vi "_UpdateCalMethod.vi"(4 "Model Name":T1=enum."IONICS 3Q 210", 5 "UsingESI1":bool=TRUE, 6 "error in (no error)":errorcluster, 7 "Q1/Q2":string="Q1", 8 "CalOption":enum32{"Positive", "Negative"}(radio), 9 "Method":T2={"Lenses"=[{"Scan Type"=0, "Scans"=1000, "Time 1"=0.0, "Time 2"=5.0, "Value 1"=400.0, "Value 2"=400.0, "Step Size"=1.0}, {"Scan Type"=0, "Scans"=1, "Time 1"=1.0, "Time 2"=1.0, "Value 1"=600.0, "Value 2"=600.0, "Step Size"=1.0}, {"Scan Type"=0, "Scans"=1, "Time 1"=1.0, "Time 2"=1.0, "Value 1"=32000.0, "Value 2"=32000.0, "Step Size"=1.0}, {"Scan Type"=0, "Scans"=1, "Time 1"=1.0, "Time 2"=1.0, "Value 1"=400.0, "Value 2"=400.0, "Step Size"=1.0}, {"Scan Type"=0, "Scans"=1, "Time 1"=1.0, "Time 2"=1.0, "Value 1"=600.0, "Value 2"=600.0, "Step Size"=1.0}, {"Scan Type"=0, "Scans"=1, "Time 1"=1.0, "Time 2"=1.0, "Value 1"=32000.0, "Value 2"=32000.0, "Step Size"=1.0}, {"Scan Type"=0, "Scans"=1, "Time 1"=1.0, "Time 2"=1.0, "Value 1"=500.0, "Value 2"=400.0, "Step Size"=1.0}, {"Scan Type"=0, "Scans"=1, "Time 1"=1.0, "Time 2"=1.0, "Value 1"=70.0, "Value 2"=80.0, "Step Size"=1.0}, {"Scan Type"=0, "Scans"=1, "Time 1"=1.0, "Time 2"=1.0, "Value 1"=80.0, "Value 2"=80.0, "Step Size"=1.0}, {"Scan Type"=0, "Scans"=1, "Time 1"=1.0, "Time 2"=1.0, "Value 1"=-1.0, "Value 2"=100.0, "Step Size"=1.0}, {"Scan Type"=0, "Scans"=1, "Time 1"=1.0, "Time 2"=1.0, "Value 1"=-2.0, "Value 2"=100.0, "Step Size"=1.0}, {"Scan Type"=0, "Scans"=1, "Time 1"=1.0, "Time 2"=1.0, "Value 1"=-3.0, "Value 2"=100.0, "Step Size"=1.0}, {"Scan Type"=0, "Scans"=1, "Time 1"=1.0, "Time 2"=1.0, "Value 1"=-4.0, "Value 2"=100.0, "Step Size"=1.0}, {"Scan Type"=0, "Scans"=1, "Time 1"=1.0, "Time 2"=1.0, "Value 1"=-15.0, "Value 2"=100.0, "Step Size"=1.0}, {"Scan Type"=0, "Scans"=1, "Time 1"=1.0, "Time 2"=1.0, "Value 1"=-4.5, "Value 2"=-9.0, "Step Size"=1.0}, {"Scan Type"=0, "Scans"=1, "Time 1"=1.0, "Time 2"=1.0, "Value 1"=0.0, "Value 2"=100.0, "Step Size"=1.0}, {"Scan Type"=0, "Scans"=1, "Time 1"=1.0, "Time 2"=1.0, "Value 1"=-100.0, "Value 2"=100.0, "Step Size"=1.0}, {"Scan Type"=0, "Scans"=1, "Time 1"=1.0, "Time 2"=1.0, "Value 1"=-50.0, "Value 2"=100.0, "Step Size"=1.0}, {"Scan Type"=0, "Scans"=1, "Time 1"=1.0, "Time 2"=1.0, "Value 1"=100.0, "Value 2"=100.0, "Step Size"=1.0}, {"Scan Type"=0, "Scans"=1, "Time 1"=1.0, "Time 2"=1.0, "Value 1"=-51.0, "Value 2"=100.0, "Step Size"=1.0}, {"Scan Type"=0, "Scans"=1, "Time 1"=1.0, "Time 2"=1.0, "Value 1"=-62.0, "Value 2"=100.0, "Step Size"=1.0}, {"Scan Type"=0, "Scans"=1, "Time 1"=1.0, "Time 2"=1.0, "Value 1"=-52.0, "Value 2"=-150.0, "Step Size"=1.0}, {"Scan Type"=0, "Scans"=1, "Time 1"=1.0, "Time 2"=1.0, "Value 1"=-100.0, "Value 2"=-200.0, "Step Size"=1.0}, {"Scan Type"=0, "Scans"=1, "Time 1"=1.0, "Time 2"=1.0, "Value 1"=15.0, "Value 2"=50.0, "Step Size"=1.0}, {"Scan Type"=0, "Scans"=1, "Time 1"=1.0, "Time 2"=1.0, "Value 1"=2000.0, "Value 2"=500.0, "Step Size"=1.0}, {"Scan Type"=0, "Scans"=1, "Time 1"=1.0, "Time 2"=1.0, "Value 1"=5500.0, "Value 2"=1000.0, "Step Size"=1.0}, {"Scan Type"=0, "Scans"=1, "Time 1"=1.0, "Time 2"=1.0, "Value 1"=420.0, "Value 2"=420.0, "Step Size"=1.0}, {"Scan Type"=0, "Scans"=1, "Time 1"=1.0, "Time 2"=1.0, "Value 1"=-420.0, "Value 2"=-420.0, "Step Size"=1.0}, {"Scan Type"=0, "Scans"=1, "Time 1"=1.0, "Time 2"=1.0, "Value 1"=420.0, "Value 2"=420.0, "Step Size"=1.0}, {"Scan Type"=0, "Scans"=1, "Time 1"=1.0, "Time 2"=1.0, "Value 1"=-420.0, "Value 2"=-420.0, "Step Size"=1.0}, {"Scan Type"=0, "Scans"=1, "Time 1"=1.0, "Time 2"=1.0, "Value 1"=600.0, "Value 2"=600.0, "Step Size"=1.0}, {"Scan Type"=0, "Scans"=1, "Time 1"=1.0, "Time 2"=1.0, "Value 1"=-600.0, "Value 2"=600.0, "Step Size"=1.0}, {"Scan Type"=0, "Scans"=1, "Time 1"=1.0, "Time 2"=1.0, "Value 1"=80.0, "Value 2"=0.9, "Step Size"=1.0}, {"Scan Type"=0, "Scans"=1, "Time 1"=1.0, "Time 2"=1.0, "Value 1"=90.0, "Value 2"=0.0, "Step Size"=1.0}, {"Scan Type"=0, "Scans"=1, "Time 1"=1.0, "Time 2"=1.0, "Value 1"=0.0, "Value 2"=0.0, "Step Size"=1.0}, {"Scan Type"=0, "Scans"=1, "Time 1"=1.0, "Time 2"=1.0, "Value 1"=0.0, "Value 2"=0.0, "Step Size"=1.0}, {"Scan Type"=0, "Scans"=1, "Time 1"=1.0, "Time 2"=1.0, "Value 1"=0.0, "Value 2"=0.0, "Step Size"=1.0}, {"Scan Type"=0, "Scans"=1, "Time 1"=1.0, "Time 2"=1.0, "Value 1"=0.0, "Value 2"=0.0, "Step Size"=1.0}, {"Scan Type"=0, "Scans"=1, "Time 1"=1.0, "Time 2"=1.0, "Value 1"=500.0, "Value 2"=0.0, "Step Size"=1.0}, {"Scan Type"=0, "Scans"=1, "Time 1"=1.0, "Time 2"=1.0, "Value 1"=0.0, "Value 2"=0.0, "Step Size"=1.0}, {"Scan Type"=0, "Scans"=1, "Time 1"=1.0, "Time 2"=1.0, "Value 1"=5850.0, "Value 2"=0.0, "Step Size"=1.0}, {"Scan Type"=0, "Scans"=1, "Time 1"=1.0, "Time 2"=1.0, "Value 1"=0.0, "Value 2"=0.0, "Step Size"=1.0}, {"Scan Type"=0, "Scans"=1, "Time 1"=1.0, "Time 2"=1.0, "Value 1"=1000.0, "Value 2"=0.0, "Step Size"=1.0}, {"Scan Type"=0, "Scans"=1, "Time 1"=1.0, "Time 2"=1.0, "Value 1"=320.0, "Value 2"=0.0, "Step Size"=1.0}, {"Scan Type"=0, "Scans"=1, "Time 1"=1.0, "Time 2"=1.0, "Value 1"=0.0, "Value 2"=0.0, "Step Size"=1.0}, {"Scan Type"=0, "Scans"=1, "Time 1"=1.0, "Time 2"=1.0, "Value 1"=0.0, "Value 2"=0.0, "Step Size"=1.0}], "Mass Ranges"=[{"Start"=54.0, "Stop"=64.0, "Step Size"=0.1, "Steps"=101, "Dwell"=10.0, "Parameters"=[], "Res"=1}, {"Start"=170.0, "Stop"=180.0, "Step Size"=0.1, "Steps"=101, "Dwell"=10.0, "Parameters"=[], "Res"=1}, {"Start"=611.0, "Stop"=621.0, "Step Size"=0.1, "Steps"=101, "Dwell"=10.0, "Parameters"=[], "Res"=1}, {"Start"=902.0, "Stop"=912.0, "Step Size"=0.1, "Steps"=101, "Dwell"=10.0, "Parameters"=[], "Res"=1}, {"Start"=1250.0, "Stop"=1260.0, "Step Size"=0.1, "Steps"=101, "Dwell"=10.0, "Parameters"=[], "Res"=1}, {"Start"=1540.0, "Stop"=1550.0, "Step Size"=0.1, "Steps"=101, "Dwell"=10.0, "Parameters"=[], "Res"=1}, {"Start"=1773.0, "Stop"=1783.0, "Step Size"=0.1, "Steps"=101, "Dwell"=10.0, "Parameters"=[], "Res"=1}, {"Start"=2005.0, "Stop"=2015.0, "Step Size"=0.1, "Steps"=101, "Dwell"=10.0, "Parameters"=[], "Res"=1}], "Acquire"=FALSE, "MCA"=FALSE, "Q1DC EN"=FALSE, "Q1 POL"=FALSE, "Q3 POL"=FALSE, "Q1 RF  EN"=TRUE, "Averaging"=FALSE, "Log Scale"=FALSE, "CPS"=TRUE, "Unit"=FALSE, "Data Path"=path "", "Run Mode"=enum."Q1 Scan", "Fixed Mass (amu)"=609.2, "Q3DC EN"=FALSE, "Q3 RF  EN"=TRUE, "Negative"=FALSE} {"Mass Ranges"."Res" items=["High/High", "Medium/Medium", "Low/Low", "High/Medium", "High/Low", "Medium/High", "Medium/Low", "Low/High", "Low/Medium"]}) -> (0 "error out":errorcluster, 3 "MethodOut":T2={"Lenses"=[{"Scan Type"=0, "Scans"=1000, "Time 1"=0.0, "Time 2"=5.0, "Value 1"=400.0, "Value 2"=400.0, "Step Size"=1.0}, {"Scan Type"=0, "Scans"=1, "Time 1"=1.0, "Time 2"=1.0, "Value 1"=600.0, "Value 2"=600.0, "Step Size"=1.0}, {"Scan Type"=0, "Scans"=1, "Time 1"=1.0, "Time 2"=1.0, "Value 1"=32000.0, "Value 2"=32000.0, "Step Size"=1.0}, {"Scan Type"=0, "Scans"=1, "Time 1"=1.0, "Time 2"=1.0, "Value 1"=400.0, "Value 2"=400.0, "Step Size"=1.0}, {"Scan Type"=0, "Scans"=1, "Time 1"=1.0, "Time 2"=1.0, "Value 1"=600.0, "Value 2"=600.0, "Step Size"=1.0}, {"Scan Type"=0, "Scans"=1, "Time 1"=1.0, "Time 2"=1.0, "Value 1"=32000.0, "Value 2"=32000.0, "Step Size"=1.0}, {"Scan Type"=0, "Scans"=1, "Time 1"=1.0, "Time 2"=1.0, "Value 1"=500.0, "Value 2"=400.0, "Step Size"=1.0}, {"Scan Type"=0, "Scans"=1, "Time 1"=1.0, "Time 2"=1.0, "Value 1"=70.0, "Value 2"=80.0, "Step Size"=1.0}, {"Scan Type"=0, "Scans"=1, "Time 1"=1.0, "Time 2"=1.0, "Value 1"=80.0, "Value 2"=80.0, "Step Size"=1.0}, {"Scan Type"=0, "Scans"=1, "Time 1"=1.0, "Time 2"=1.0, "Value 1"=-1.0, "Value 2"=100.0, "Step Size"=1.0}, {"Scan Type"=0, "Scans"=1, "Time 1"=1.0, "Time 2"=1.0, "Value 1"=-2.0, "Value 2"=100.0, "Step Size"=1.0}, {"Scan Type"=0, "Scans"=1, "Time 1"=1.0, "Time 2"=1.0, "Value 1"=-3.0, "Value 2"=100.0, "Step Size"=1.0}, {"Scan Type"=0, "Scans"=1, "Time 1"=1.0, "Time 2"=1.0, "Value 1"=-4.0, "Value 2"=100.0, "Step Size"=1.0}, {"Scan Type"=0, "Scans"=1, "Time 1"=1.0, "Time 2"=1.0, "Value 1"=-15.0, "Value 2"=100.0, "Step Size"=1.0}, {"Scan Type"=0, "Scans"=1, "Time 1"=1.0, "Time 2"=1.0, "Value 1"=-4.5, "Value 2"=-9.0, "Step Size"=1.0}, {"Scan Type"=0, "Scans"=1, "Time 1"=1.0, "Time 2"=1.0, "Value 1"=0.0, "Value 2"=100.0, "Step Size"=1.0}, {"Scan Type"=0, "Scans"=1, "Time 1"=1.0, "Time 2"=1.0, "Value 1"=-100.0, "Value 2"=100.0, "Step Size"=1.0}, {"Scan Type"=0, "Scans"=1, "Time 1"=1.0, "Time 2"=1.0, "Value 1"=-50.0, "Value 2"=100.0, "Step Size"=1.0}, {"Scan Type"=0, "Scans"=1, "Time 1"=1.0, "Time 2"=1.0, "Value 1"=100.0, "Value 2"=100.0, "Step Size"=1.0}, {"Scan Type"=0, "Scans"=1, "Time 1"=1.0, "Time 2"=1.0, "Value 1"=-51.0, "Value 2"=100.0, "Step Size"=1.0}, {"Scan Type"=0, "Scans"=1, "Time 1"=1.0, "Time 2"=1.0, "Value 1"=-62.0, "Value 2"=100.0, "Step Size"=1.0}, {"Scan Type"=0, "Scans"=1, "Time 1"=1.0, "Time 2"=1.0, "Value 1"=-52.0, "Value 2"=-150.0, "Step Size"=1.0}, {"Scan Type"=0, "Scans"=1, "Time 1"=1.0, "Time 2"=1.0, "Value 1"=-100.0, "Value 2"=-200.0, "Step Size"=1.0}, {"Scan Type"=0, "Scans"=1, "Time 1"=1.0, "Time 2"=1.0, "Value 1"=15.0, "Value 2"=50.0, "Step Size"=1.0}, {"Scan Type"=0, "Scans"=1, "Time 1"=1.0, "Time 2"=1.0, "Value 1"=2000.0, "Value 2"=500.0, "Step Size"=1.0}, {"Scan Type"=0, "Scans"=1, "Time 1"=1.0, "Time 2"=1.0, "Value 1"=5500.0, "Value 2"=1000.0, "Step Size"=1.0}, {"Scan Type"=0, "Scans"=1, "Time 1"=1.0, "Time 2"=1.0, "Value 1"=420.0, "Value 2"=420.0, "Step Size"=1.0}, {"Scan Type"=0, "Scans"=1, "Time 1"=1.0, "Time 2"=1.0, "Value 1"=-420.0, "Value 2"=-420.0, "Step Size"=1.0}, {"Scan Type"=0, "Scans"=1, "Time 1"=1.0, "Time 2"=1.0, "Value 1"=420.0, "Value 2"=420.0, "Step Size"=1.0}, {"Scan Type"=0, "Scans"=1, "Time 1"=1.0, "Time 2"=1.0, "Value 1"=-420.0, "Value 2"=-420.0, "Step Size"=1.0}, {"Scan Type"=0, "Scans"=1, "Time 1"=1.0, "Time 2"=1.0, "Value 1"=600.0, "Value 2"=600.0, "Step Size"=1.0}, {"Scan Type"=0, "Scans"=1, "Time 1"=1.0, "Time 2"=1.0, "Value 1"=-600.0, "Value 2"=600.0, "Step Size"=1.0}, {"Scan Type"=0, "Scans"=1, "Time 1"=1.0, "Time 2"=1.0, "Value 1"=80.0, "Value 2"=0.9, "Step Size"=1.0}, {"Scan Type"=0, "Scans"=1, "Time 1"=1.0, "Time 2"=1.0, "Value 1"=90.0, "Value 2"=0.0, "Step Size"=1.0}, {"Scan Type"=0, "Scans"=1, "Time 1"=1.0, "Time 2"=1.0, "Value 1"=0.0, "Value 2"=0.0, "Step Size"=1.0}, {"Scan Type"=0, "Scans"=1, "Time 1"=1.0, "Time 2"=1.0, "Value 1"=0.0, "Value 2"=0.0, "Step Size"=1.0}, {"Scan Type"=0, "Scans"=1, "Time 1"=1.0, "Time 2"=1.0, "Value 1"=0.0, "Value 2"=0.0, "Step Size"=1.0}, {"Scan Type"=0, "Scans"=1, "Time 1"=1.0, "Time 2"=1.0, "Value 1"=0.0, "Value 2"=0.0, "Step Size"=1.0}, {"Scan Type"=0, "Scans"=1, "Time 1"=1.0, "Time 2"=1.0, "Value 1"=500.0, "Value 2"=0.0, "Step Size"=1.0}, {"Scan Type"=0, "Scans"=1, "Time 1"=1.0, "Time 2"=1.0, "Value 1"=0.0, "Value 2"=0.0, "Step Size"=1.0}, {"Scan Type"=0, "Scans"=1, "Time 1"=1.0, "Time 2"=1.0, "Value 1"=5850.0, "Value 2"=0.0, "Step Size"=1.0}, {"Scan Type"=0, "Scans"=1, "Time 1"=1.0, "Time 2"=1.0, "Value 1"=0.0, "Value 2"=0.0, "Step Size"=1.0}, {"Scan Type"=0, "Scans"=1, "Time 1"=1.0, "Time 2"=1.0, "Value 1"=1000.0, "Value 2"=0.0, "Step Size"=1.0}, {"Scan Type"=0, "Scans"=1, "Time 1"=1.0, "Time 2"=1.0, "Value 1"=320.0, "Value 2"=0.0, "Step Size"=1.0}, {"Scan Type"=0, "Scans"=1, "Time 1"=1.0, "Time 2"=1.0, "Value 1"=0.0, "Value 2"=0.0, "Step Size"=1.0}, {"Scan Type"=0, "Scans"=1, "Time 1"=1.0, "Time 2"=1.0, "Value 1"=0.0, "Value 2"=0.0, "Step Size"=1.0}], "Mass Ranges"=[{"Start"=54.0, "Stop"=64.0, "Step Size"=0.1, "Steps"=101, "Dwell"=10.0, "Parameters"=[], "Res"=1}, {"Start"=170.0, "Stop"=180.0, "Step Size"=0.1, "Steps"=101, "Dwell"=10.0, "Parameters"=[], "Res"=1}, {"Start"=611.0, "Stop"=621.0, "Step Size"=0.1, "Steps"=101, "Dwell"=10.0, "Parameters"=[], "Res"=1}, {"Start"=902.0, "Stop"=912.0, "Step Size"=0.1, "Steps"=101, "Dwell"=10.0, "Parameters"=[], "Res"=1}, {"Start"=1250.0, "Stop"=1260.0, "Step Size"=0.1, "Steps"=101, "Dwell"=10.0, "Parameters"=[], "Res"=1}, {"Start"=1540.0, "Stop"=1550.0, "Step Size"=0.1, "Steps"=101, "Dwell"=10.0, "Parameters"=[], "Res"=1}, {"Start"=1773.0, "Stop"=1783.0, "Step Size"=0.1, "Steps"=101, "Dwell"=10.0, "Parameters"=[], "Res"=1}, {"Start"=2005.0, "Stop"=2015.0, "Step Size"=0.1, "Steps"=101, "Dwell"=10.0, "Parameters"=[], "Res"=1}], "Acquire"=FALSE, "MCA"=FALSE, "Q1DC EN"=FALSE, "Q1 POL"=FALSE, "Q3 POL"=FALSE, "Q1 RF  EN"=TRUE, "Averaging"=FALSE, "Log Scale"=FALSE, "CPS"=TRUE, "Unit"=FALSE, "Data Path"=path "", "Run Mode"=enum."Q1 Scan", "Fixed Mass (amu)"=609.2, "Q3DC EN"=FALSE, "Q3 RF  EN"=TRUE, "Negative"=FALSE} {"Mass Ranges"."Res" items=["High/High", "Medium/Medium", "Low/Low", "High/Medium", "High/Low", "Medium/High", "Medium/Low", "Low/High", "Low/Medium"]})   [LabVIEW 2012]
uses:
  Type/_GUI Method.ctl
  Type/_Lens Property.ctl
  Type/_Mass Range Property.ctl
  Type/_Mass Range Parameters.ctl
  Type/_RT Res Type.ctl
  Type/_Run Mode.ctl
  Type/_Instrument Model.ctl
panel:
  in  "CurrentDV":dbl=2000.0
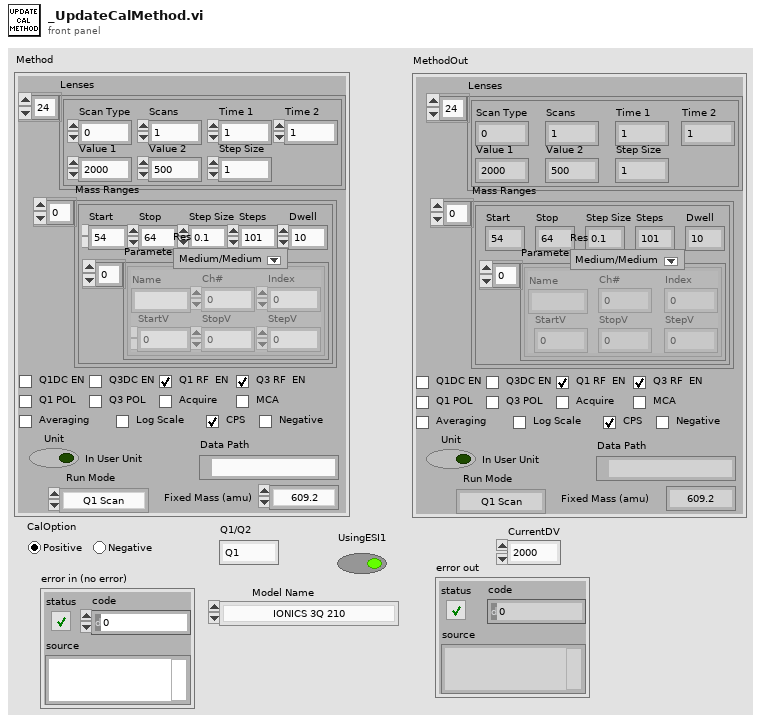
[diagram p1: front panel]
types:
  T1 = typedef "_Instrument Model.ctl" = enum16{"IONICS 3QA", "IONICS 3QB", "IONICS 3Q 110", "IONICS 3Q 120", "IONICS 3Q 210", "IONICS 3Q 220", "IONICS 3Q 310", "IONICS 3Q 320", "SHIMADZU LCMS-8080", "Simulation (Single Source)", "Simulation (Dual Source)"}
  T2 = typedef "_GUI Method.ctl" = cluster{"Lenses":T3[], "Mass Ranges":T4[], "Acquire":bool, "MCA":bool, "Q1DC EN":bool, "Q1 POL":bool, "Q3 POL":bool, "Q1 RF  EN":bool, "Averaging":bool, "Log Scale":bool, "CPS":bool, "Unit":bool, "Data Path":path, "Run Mode":T7, "Fixed Mass (amu)":dbl, "Q3DC EN":bool, "Q3 RF  EN":bool, "Negative":bool}
  T3 = typedef "_Lens Property.ctl" = cluster{"Scan Type":u8, "Scans":i32, "Time 1":dbl, "Time 2":dbl, "Value 1":dbl, "Value 2":dbl, "Step Size":dbl}
  T4 = typedef "_Mass Range Property.ctl" = cluster{"Start":dbl, "Stop":dbl, "Step Size":dbl, "Steps":i32, "Dwell":dbl, "Parameters":T5[], "Res":T6}
  T5 = typedef "_Mass Range Parameters.ctl" = cluster{"Name":string, "Ch#":u8, "StartV":dbl, "StopV":dbl, "StepV":dbl, "Index":u8}
  T6 = typedef "_RT Res Type.ctl" = u16
  T7 = typedef "_Run Mode.ctl" = enum16{"MRM (Q1/Q2)", "Q1 Scan", "Q1 SRM", "Q2 Scan", "Q2 SRM", "Product Scan", "Precursor Scan", "Neutral Loss", "Neutral Gain"}
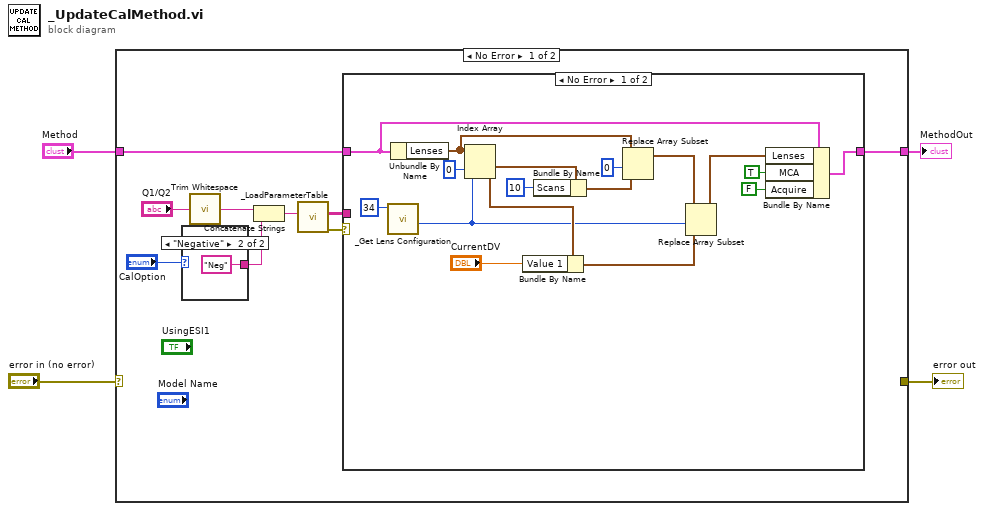
[diagram p0: block diagram]
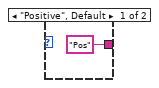
[diagram p3: hidden frame]
diagram:
  n1 = case shown="No Error" "error in (no error)" {
    selector: "error in (no error)" -> [_ w34]
    tunnel: "Method" -> [w13 w35]
    tunnel: [w12 w35] -> w3
    tunnel: [_ w34] -> w1
    frame No Error {
      n2 = case shown="\"Negative\"" "CalOption" {
        tunnel: ["Pos" "Neg"] -> w8
        frame "Positive", Default {
        }
        frame "Negative" {
        }
      }
      n3 = call <vilib>:"Trim Whitespace.vi"("string"="Q1/Q2") -> ("trimmed string"=w9:string)  [unwired: 1 in]
      n4 = Concatenate Strings(w9, w8) -> (w7:string)
      n5 = call "_LoadParameterTable.vi"("ScanMode"=w7) -> ("error out"=w6:errorcluster, "ParameterList"=w5:string[][])  [unwired: 5 in]
      n6 = case shown="No Error" w6 {
        tunnel: w13 -> [w24 w31]
        tunnel: [w14 w31] -> w12
        tunnel: w5 -> [_ _]
        frame No Error {
          n7 = call "_Get Lens Configuration.vi"("Channel #"=u8 34) -> ("Config Row#"=w18:i32)  [unwired: 1 in, 5 out]
          n8 = Unbundle By Name(w24) -> ("Lenses"=w27:T3[])
          n9 = Index Array(array=w27, index #1=0 ("index"), index #2=w18) -> (element #1=w29:T3, element #2=w20:T3)
          n10 = Bundle By Name(cluster=w20, "Value 1"="CurrentDV") -> (w17:T3)
          n11 = Bundle By Name(cluster=w29, "Scans"=10) -> (w25:T3)
          n12 = Replace Array Subset(array=w27, new element=w25, index=0) -> (w16:T3[])
          n13 = Replace Array Subset(array=w16, new element=w17, index=w18) -> (w15:T3[])
          n14 = Bundle By Name(cluster=w24, "Lenses"=w15, "MCA"=TRUE, "Acquire"=FALSE) -> (w14:T2)
        }
        frame Error {
          # "Parameter table cannot be loaded, the cal method was not modified\nbut this error is ignored as we proceed with the default method."
        }
      }
    }
    frame Error {
    }
  }
  "MethodOut" <- w3
  "error out" <- w1
